vi "Photon Counter Reader.vi"(8 "error in (no error)":errorcluster, 10 "Photon Counter in":refnum<class "Photon Counter.lvclass">, 11 "PC Reader in":refnum<class "Photon Counter Reader.lvclass">) -> (0 "error out":errorcluster, 3 "PC Reader out":refnum<class "Photon Counter Reader.lvclass">)   [LabVIEW 2017, in "Photon Counter Reader.lvclass"]
uses:
  Photon Counter Reader.lvclass
  C:/LabVIEW-programs/Readers/Reader/Reader.lvclass
  Instruments/Photon Counter/Photon Counter.lvclass
  C:/LabVIEW-programs/Instruments/Utility Classes/Readable/Readable.lvclass
  Reader/Reader.lvclass
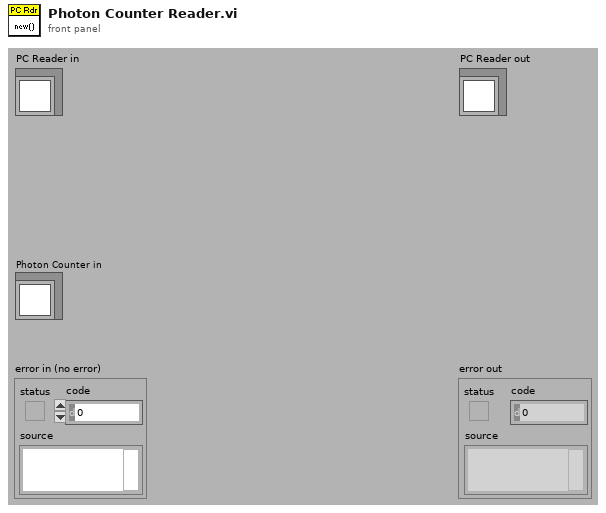
[diagram p1: front panel]
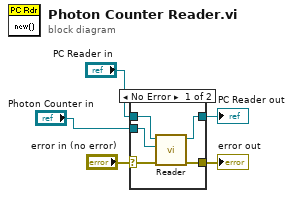
[diagram p0: block diagram]
diagram:
  n1 = case shown="No Error" "error in (no error)" {
    selector: "error in (no error)" -> [w9 w12]
    tunnel: [w8 w12] -> w4
    tunnel: [w6 w11] -> w2
    tunnel: "PC Reader in" -> [w10 w11]
    tunnel: "Photon Counter in" -> [w7 _]
    frame No Error {
      n2 = call "Reader.vi"("error in (no error)"=w9, "Readable"=w7, "Reader in"=w10) -> ("error out"=w8:errorcluster, "Reader out"=w6:refnum<class "Photon Counter Reader.lvclass">)  [unwired: 7 out]
    }
    frame Error {
    }
  }
  "error out" <- w4
  "PC Reader out" <- w2
